vi "test - docs pure English.vi"(8 "error in (no error)":errorcluster, 11 "TestCase in":refnum<class "testcase-documentation.lvclass">) -> (0 "error out":errorcluster, 3 "TestCase out":refnum<class "testcase-documentation.lvclass">)   [LabVIEW 2017, in "testcase-documentation.lvclass"]
uses:
  testcase-documentation.lvclass
  <vilib>/addons/_JKI Toolkits/VI Tester/TestCase.llb/TestCase.lvclass
  src/user.lib/_NEVSTOP/Communicable State Machine(CSM)/_csmDoc/csmdoc.lvlib
  src/user.lib/_NEVSTOP/Communicable State Machine(CSM)/_Shared/CSM Shared.lvlib
  src/user.lib/_NEVSTOP/Communicable State Machine(CSM)/Communicable State Machine.lvlib
  C:/Program Files (x86)/National Instruments/LabVIEW 2017/vi.lib/addons/_JKI Toolkits/VI Tester/TestCase.llb/TestCase.lvclass
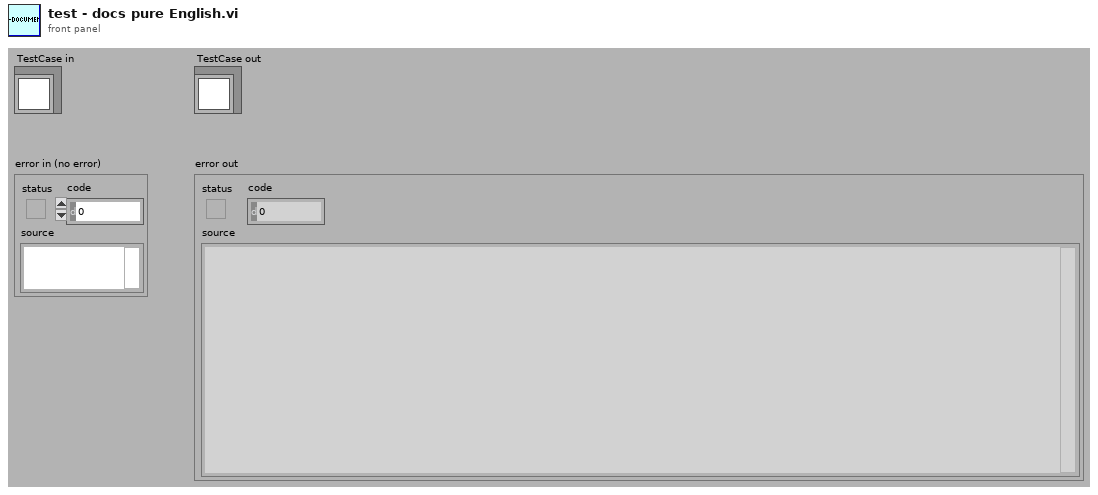
[diagram p1: front panel]
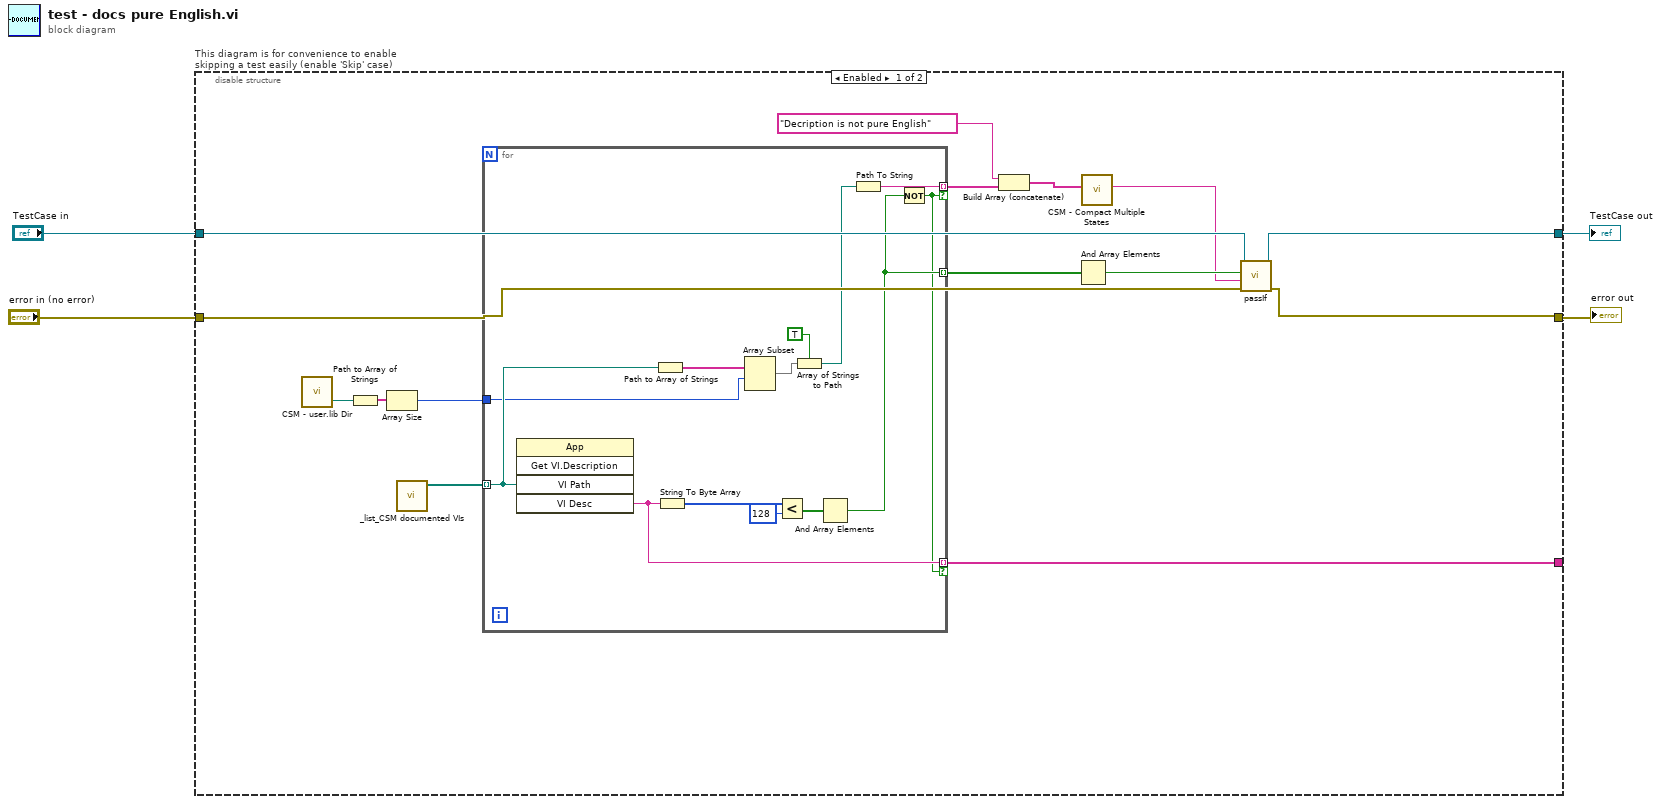
[diagram p0: block diagram]
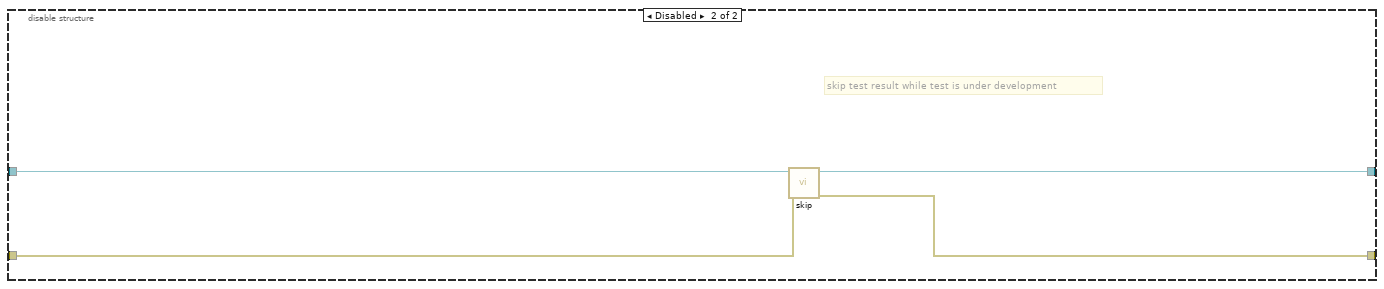
[diagram p2: hidden frame]
diagram:
  n1 = disable-structure "This diagram is for convenience to enable skipping a test easily (enable 'Skip' case)" shown="Enabled" {
    disable-tunnel: "TestCase in" -> [w19 w36]
    disable-tunnel: [w18 w34] -> w1
    disable-tunnel: [w17 w35] -> w3
    disable-tunnel: "error in (no error)" -> [w16 w33]
    disable-tunnel: [w5 _] -> _
    frame Enabled {
      n2 = call "CSM - user.lib Dir.vi"() -> ("<LabVIEW>"=w13:path)  [unwired: 2 in, 1 out]
      n3 = Path to Array of Strings(0:w13) -> (2:w14:string[])  [unwired: 1 out]
      n4 = Array Size(array=w14) -> (size(s)=w12:i32)
      n5 = call "_list_CSM documented VIs.vi"() -> ("Array"=w15:path[])  [unwired: 11 in]
      n6 = for {
        tunnel: w15 -> [w32] mode=indexing
        tunnel: w12 -> [w31]
        tunnel: [w22] -> w11 mode=indexing
        tunnel: [w27] -> w10 mode=indexing if=w20
        tunnel: [w21] -> w5 mode=indexing if=w20
        n7 = invoke class="App" method="Get VI.Description"("VI Path"=w32) -> ("VI Desc"=w21:string)  [unwired: 4 in, 4 out]
        n8 = Path to Array of Strings(0:w32) -> (2:w24:string[])  [unwired: 1 out]
        n9 = String To Byte Array(string=w21) -> (unsigned byte array=w30:u8[])
        n10 = Array Subset(array=w24, index=w31) -> (w26:string[])  [unwired: 1 in]
        n11 = Less?(x=w30, y=u8 128) -> (x < y?=w28:bool[])
        n12 = Array of Strings to Path(0:w26, 1:TRUE ("relative")) -> (2:w23:path)
        n13 = And Array Elements(Boolean array=w28) -> (logical AND=w22:bool)
        n14 = Path To String(path=w23) -> (string=w27:string)
        n15 = Not(x=w22) -> (.not. x?=w20:bool)
      }
      n16 = Build Array (concatenate)("Decription is not pure English" ("message (\"\")"), w10) -> (w8:string[])
      n17 = And Array Elements(Boolean array=w11) -> (logical AND=w9:bool)
      n18 = call "CSM - Compact Multiple States.vi"("Multiple States"=w8) -> ("States"=w6:string)  [unwired: 9 in]
      n19 = call-dynamic "passIf.vi"("error in (no error)"=w16, "message (\"\")"=w6, "pass"=w9, "TestCase in"=w19) -> ("error out"=w17:errorcluster, "TestCase out"=w18:refnum<class "testcase-documentation.lvclass">)  [unwired: 6 in]
    }
    frame Disabled {
      # "skip test result while test is under development"
      n20 = call <vilib>:"skip.vi"("error in (no error)"=w33, "TestCase in"=w36) -> ("error out"=w35:errorcluster, "TestCase out"=w34:refnum<class "testcase-documentation.lvclass">)  [unwired: 8 in]
    }
  }
  "error out" <- w3
  "TestCase out" <- w1
